vi "Close old and open new AVI file.vi"(8 "error in (no error)":errorcluster, 10 "AVI File Path":path, 11 "AVI modes refs":T1) -> (0 "error out":errorcluster, 1 "Number of Frames":u32, 2 "Cancelled due to the selected \nAVI file being located within an\n\"Exported 8-bit videos\" directory!":bool, 3 "AVI modes refs":T1, 5 "Reinitialising in AVI1 mode":bool)   [LabVIEW 2017]
uses:
  Typedefs/AVI modes refs cluster.ctl
  <vilib>/vision/Avi1.llb/AviRefnum.ctl
  <vilib>/vision/Avi.llb/IMAQ AVI2 Refnum.ctl
  Globals/gl_Time series viewer globals.vi
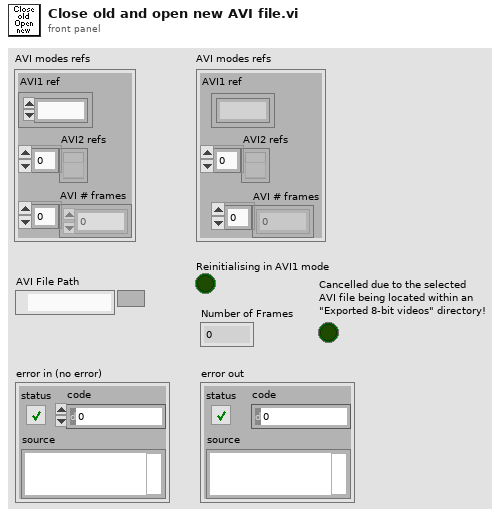
[diagram p1: front panel]
types:
  T1 = typedef "AVI modes refs cluster.ctl" = cluster{"AVI1 ref":T2, "AVI2 refs":T3[], "AVI # frames":u32[]}
  T2 = typedef "AviRefnum.ctl" = refnum<k1>
  T3 = typedef "IMAQ AVI2 Refnum.ctl" = refnum<k20>
  T4 = typedef "AVI implementation enum.ctl" = enum16{"AVI1", "AVI2"}
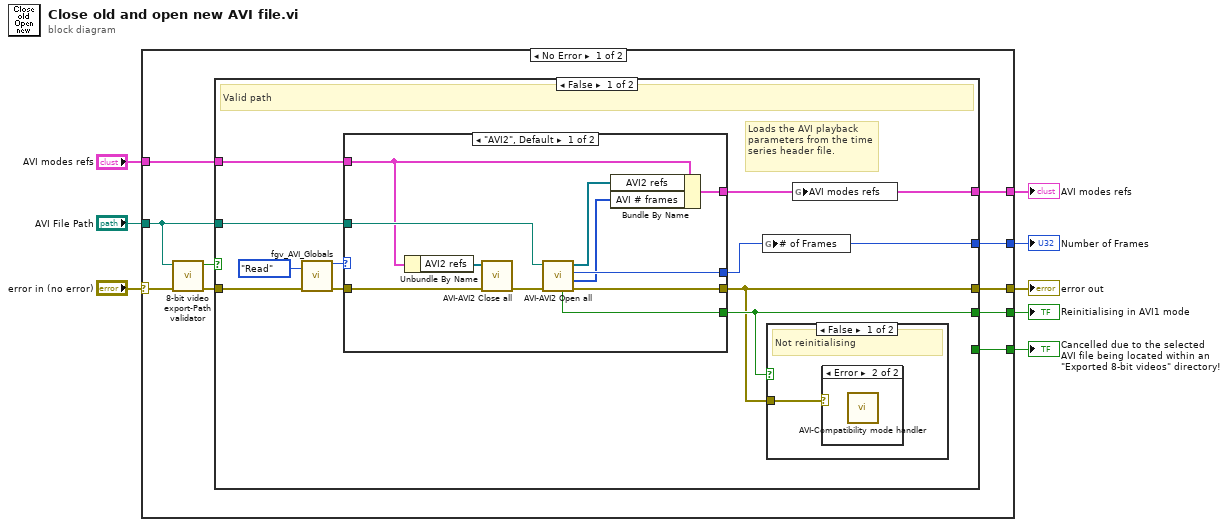
[diagram p0: block diagram]
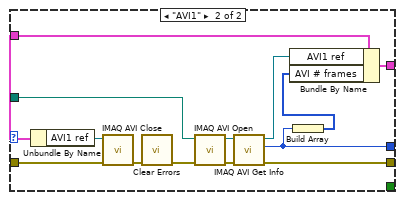
[diagram p4: hidden frame]
diagram:
  n1 = case shown="No Error" "error in (no error)" {
    selector: "error in (no error)" -> [w12 w57]
    tunnel: "AVI File Path" -> [w13 _]
    tunnel: "AVI modes refs" -> [w18 w56]
    tunnel: [w14 w56] -> w6
    tunnel: [w15 w57] -> w5
    tunnel: [w17 _] -> w4
    tunnel: [w16 _] -> w2
    tunnel: [w9 _] -> w1
    frame No Error {
      n2 = call "8-bit video export-Path validator.vi"("error in (no error)"=w12, "AVI File Path"=w13) -> ("error out"=w11:errorcluster, "Invalid folder"=w10:bool)  [unwired: 8 in]
      n3 = case shown="False" w10 {
        selector: w10 -> [_ w54]
        tunnel: w18 -> [w28 w55]
        tunnel: [w25 _] -> w17
        tunnel: [w23 _] -> w16
        tunnel: [w22 _] -> w15
        tunnel: [w21 w55] -> w14
        tunnel: w13 -> [w20 _]
        tunnel: w11 -> [w19 _]
        tunnel: [_ w54] -> w9
        frame False {
          # "Loads the AVI playback parameters from the time series header file."
          # "Valid path"
          n4 = call "fgv_AVI_Globals.vi"("Function"=enum16{"Intialize", "Write", "Read", "Clear"}."Read", "error in (no error)"=w19) -> ("AVI mode"=w26:T4, "error out"=w24:errorcluster)  [unwired: 10 in, 2 out]
          n5 = case shown="\"AVI2\", Default" w26 {
            tunnel: [w36 w42] -> w25
            tunnel: w20 -> [w37 w44]
            tunnel: [w39 w53] -> w22
            tunnel: w28 -> [w32 w47]
            tunnel: [w40 w45] -> w21
            tunnel: w24 -> [w34 w43]
            tunnel: [w30 _] -> w23
            frame "AVI2", Default {
              n6 = Unbundle By Name(w32) -> ("AVI2 refs"=w33:T3[])
              n7 = call "AVI-AVI2 Close all.vi"("error in (no error)"=w34, "AVI2 ref"=w33) -> ("error out"=w35:errorcluster)  [unwired: 9 in]
              n8 = call "AVI-AVI2 Open all.vi"("error in (no error)"=w35, "First AVI2 video's Path"=w37) -> ("error out"=w39:errorcluster, "Number of frames in each AVI2 file"=w31:u32[], "Number of Frames (across all split videos)"=w36:u32, "AVI2 split file refs"=w38:T3[], "Reinitialising in AVI1 mode"=w30:bool)  [unwired: 5 in]
              n9 = Bundle By Name(cluster=w32, "AVI2 refs"=w38, "AVI # frames"=w31) -> (w40:T1)
            }
            frame "AVI1" {
              n10 = Unbundle By Name(w47) -> ("AVI1 ref"=w49:T2)
              n11 = call "IMAQ AVI Close"("error in (no error)"=w43, "Avi Refnum"=w49) -> ("error out"=w50:errorcluster)  [unwired: 9 in]
              n12 = call <vilib>:"Clear Errors.vi"("error in (no error)"=w50) -> ("error out"=w48:errorcluster)  [unwired: 5 in, 1 out]
              n13 = call "IMAQ AVI Open"("error in (no error)"=w48, "AVI Path"=w44) -> ("error out"=w52:errorcluster, "Avi Refnum"=w51:T2)  [unwired: 8 in]
              n14 = call "IMAQ AVI Get Info"("error in (no error)"=w52, "Avi Refnum"=w51) -> ("error out"=w53:errorcluster, "Number of Frames"=w42:u32, "Avi Refnum (duplicate)"=w46:T2)  [unwired: 5 in, 2 out]
              n15 = Build Array(w42) -> (w41:u32[])
              n16 = Bundle By Name(cluster=w47, "AVI1 ref"=w46, "AVI # frames"=w41) -> (w45:T1)
            }
          }
          n17 = global write "gl_Time series viewer globals.vi" "# of Frames"(w25) -> ()
          n18 = case shown="False" w23 {
            tunnel: w22 -> [w29 _]
            frame False {
              # "Not reinitialising"
              n19 = case shown="Error" w29 {
                frame No Error {
                }
                frame Error {
                  n20 = call "AVI-Compatibility mode handler.vi"() -> ()  [unwired: 11 in, 1 out]
                }
              }
            }
            frame True {
              # "Reinitialising in AVI1 mode"
            }
          }
          n21 = global write "gl_Time series viewer globals.vi" "AVI modes refs"(w21) -> ()
        }
        frame True {
          # "Invalid path / The selected video file exists inside an \"Exported 8-bit videos\" directory."
        }
      }
    }
    frame Error {
    }
  }
  "error out" <- w5
  "Number of Frames" <- w4
  "AVI modes refs" <- w6
  "Reinitialising in AVI1 mode" <- w2
  "Cancelled due to the selected \nAVI file being located within an\n\"Exported 8-bit videos\" directory!" <- w1
